vi "main.vi"(11 "Message In":T1) -> (5 "Message Out":T1)   [LabVIEW 2025, in "Module 2.lvlib"]
uses:
  Module 2.lvlib
  <extravilib>/ChannelInstances/Event Messenger-c(str,var)/))Channel.ctl
  9e34eda5-381a-4d80-aa95-b7e8061caea7.vi
  b5b7d6df-1c06-4f02-a7d2-e48fba7cbefd.vi
  <vilib>/Utility/error.llb/Clear Errors.vi
  <extravilib>/ChannelInstances/Event Messenger-c(str,var)/))Channel.vi
  <extravilib>/ChannelInstances/Event Messenger-c(str,var)/Instantiate.vi
  Channel Messages/9242 error converting cmd string to case enum--error.vi
  Channel Messages/Bundle Module Message/Bundle Module Message.xnode
  <extravilib>/ChannelInstances/Event Messenger-c(str,var).lvlib
panel:
  in  "Log Button":bool
  in  "Log Text":string
  in  "module_interface":map{string, variant}(c390)={"Kill"=variant, "Sum"=variant(cluster{"summand0":dbl, "summand1":dbl} {"summand0"=0.0, "summand1"=0.0}), "_Log"=variant(string "")}
  out "log":string
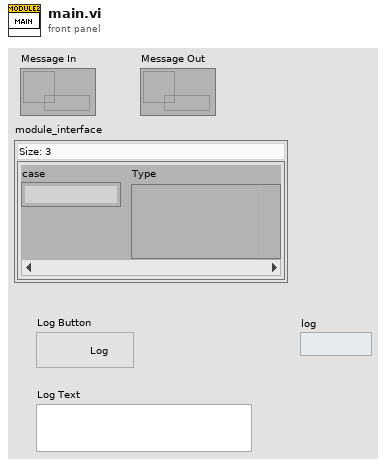
[diagram p1: front panel]
types:
  T1 = typedef "Event Messenger-c(str,var).lvlib/))Channel.ctl" = refnum<queue>
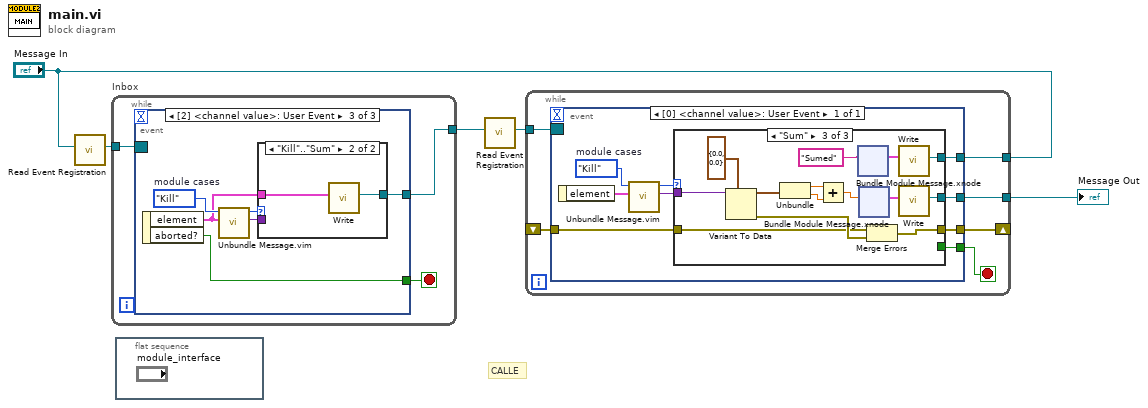
[diagram p0: block diagram]
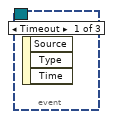
[diagram p2: hidden frame]
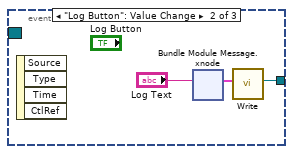
[diagram p3: hidden frame]
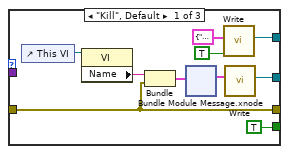
[diagram p5: hidden frame]
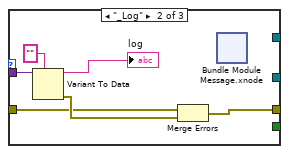
[diagram p6: hidden frame]
diagram:
  # "CALLE"
  n1 = call <extravilib>:"Read Event Registration.vi"("channel"="Message In") -> ("event registration refnum"=w3:refnum<event-registration>)  [unwired: 10 in]
  n2 = while "Inbox" {
    tunnel: [w8] -> w5
    tunnel: w3 -> [w7]
    stop <- w6 stop-if-true
    n3 = event shown="[2] <channel value>: User Event" {
      selector: w7 -> [_ _ _]
      dyn-events: _ -> [_ _ _]
      timeout: _ -> [_ _ _]
      tunnel: [_ w11 w19] -> w8
      tunnel: [_ _ w17] -> w6
      event Timeout {
        n4 = event-data() -> ()  [unwired: 1 in, 3 out]
      }
      event "Log Button": Value Change {
        n5 = event-data() -> ()  [unwired: 1 in, 4 out]
        n6 = xnode "Bundle Module Message.xnode"("data"="Log Text") -> ("message"=w10:cluster{"cmd":string, "data":variant})  [unwired: 1 in, 1 out]
        n7 = call <extravilib>:"Write.vi"("element"=w10) -> ("channel"=w11:T1)  [unwired: 9 in, 1 out]
      }
      event User Event {
        w22 = enum16{"Kill", "_Log", "Sum"}."Kill"  # module cases
        n8 = event-data() -> ("element"=w18:cluster{"cmd":string, "data":variant}, "aborted?"=w17:bool)  [unwired: 1 in]
        n9 = call "Unbundle Message.vim"("message"=w18, "case type"=w22) -> ("data"=w20:variant, "case"=w21:enum16{"Kill", "_Log", "Sum"})  [unwired: 7 in, 1 out]
        n10 = case shown="\"Kill\"..\"Sum\"" w21 {
          tunnel: w20 -> [_ _]
          tunnel: [_ w23] -> w19
          tunnel: w18 -> [_ w24]
          frame Default {
          }
          frame "Kill".."Sum" {
            n11 = call <extravilib>:"Write.vi"("element"=w24) -> ("channel"=w23:T1)  [unwired: 9 in, 1 out]
          }
        }
      }
    }
  }
  n12 = flat-sequence {
    frame #0 {
    }
  }
  n13 = call <extravilib>:"Read Event Registration.vi"("channel"=w5) -> ("event registration refnum"=w4:refnum<event-registration>)  [unwired: 10 in]
  n14 = while {
    tunnel: w4 -> [w30]
    tunnel: "Message In" -> [w27]
    shift-right: [w29] -> _
    shift-left: _ -> [w26]
    tunnel: [w25] -> w1
    stop <- w28 stop-if-true
    n15 = event shown="[0] <channel value>: User Event" {
      selector: w30 -> [_]
      dyn-events: _ -> [_]
      timeout: _ -> [_]
      tunnel: [w39] -> w29
      tunnel: [w38] -> w28
      tunnel: [w31] -> w27
      tunnel: w26 -> [w33]
      tunnel: [w32] -> w25
      event User Event {
        w34 = enum16{"Kill", "_Log", "Sum"}."Kill"  # module cases
        n16 = event-data() -> ("element"=w37:cluster{"cmd":string, "data":variant})  [unwired: 1 in]
        n17 = call "Unbundle Message.vim"("message"=w37, "case type"=w34) -> ("data"=w36:variant, "case"=w35:enum16{"Kill", "_Log", "Sum"})  [unwired: 7 in, 1 out]
        n18 = case shown="\"Sum\"" w35 {
          tunnel: w36 -> [_ w58 w79]
          tunnel: [w43 w56 w73] -> w39
          tunnel: [TRUE _ _] -> w38
          tunnel: w33 -> [w43 w55 w72]
          tunnel: [w48 _ w70] -> w32
          tunnel: [w42 _ w67] -> w31
          frame "Kill", Default {
            n19 = control-ref of="This VI"() -> (w46:refnum<vi>)
            n20 = property class="VI"(reference=w46) -> ("Name"=w45:string)  [unwired: 1 in, 2 out]
            n21 = Bundle("Name"=w45, "error IO"=w43) -> (w44:cluster{"Name":string, "error IO":errorcluster})  [unwired: 1 in]
            n22 = xnode "Bundle Module Message.xnode"("data"=w44) -> ("message"=w47:cluster{"cmd":string, "data":variant})  [unwired: 1 in, 1 out]
            n23 = call <extravilib>:"Write.vi"("abort (F)"=TRUE, "element"=cluster{"cmd":string, "data":variant} {"cmd"="", "data"=variant}) -> ("channel"=w42:T1)  [unwired: 8 in, 1 out]
            n24 = call <extravilib>:"Write.vi"("element"=w47) -> ("channel"=w48:T1)  [unwired: 9 in, 1 out]
          }
          frame "_Log" {
            n25 = Variant To Data(type="", Variant=w58) -> (data=→"log":string, error out=w57:errorcluster)  [unwired: 1 in]
            n26 = Merge Errors(w55, w57) -> (w56:errorcluster)
            n27 = xnode "Bundle Module Message.xnode"() -> ()  [unwired: 2 in, 2 out]
          }
          frame "Sum" {
            n28 = Variant To Data(type=cluster{"summand0":dbl, "summand1":dbl} {"summand0"=0.0, "summand1"=0.0} ("summands"), Variant=w79) -> (data=w77:cluster{"summand0":dbl, "summand1":dbl}, error out=w74:errorcluster)  [unwired: 1 in]
            n29 = Unbundle(w77) -> ("summand0"=w76:dbl, "summand1"=w75:dbl)
            n30 = Add(x=w76, y=w75) -> (x+y=w69:dbl)
            n31 = xnode "Bundle Module Message.xnode"("data"="Sumed") -> ("message"=w68:cluster{"cmd":string, "data":variant})  [unwired: 1 in, 1 out]
            n32 = xnode "Bundle Module Message.xnode"("data"=w69) -> ("message"=w71:cluster{"cmd":string, "data":variant})  [unwired: 1 in, 1 out]
            n33 = Merge Errors(w72, w74) -> (w73:errorcluster)
            n34 = call <extravilib>:"Write.vi"("element"=w68) -> ("channel"=w67:T1)  [unwired: 9 in, 1 out]
            n35 = call <extravilib>:"Write.vi"("element"=w71) -> ("channel"=w70:T1)  [unwired: 9 in, 1 out]
          }
        }
      }
    }
  }
  "Message Out" <- w1
